vi "SVD_ImagePerEig.vi"(0 "frame":i32, 6 "first N index":i32, 8 "output cluster":T2, 10 "Index Order":dbl[](array[numeric]), 11 "Input Casarati":cdb[][](array[numeric])) -> (2 "StackedImages":cdb[][][](array[numeric]))   [LabVIEW 2022 SP3]
uses:
  <vilib>/Analysis/Matrix/Datatypes/ComplexMatrix.ctl
  <vilib>/Analysis/7linalg.llb/Complex Conjugate Transpose Matrix.vi
  <vilib>/Analysis/baseanly.llb/Complex Outer Product.vi
  <vilib>/Analysis/baseanly.llb/Complex A x B.vi
  <vilib>/Analysis/Matrix/Numeric/Conversions/Matrix To Array - CM.vi
  <vilib>/Analysis/NI_AALPro.lvlib
  <vilib>/Analysis/NI_AALBase.lvlib
  <vilib>/Analysis/Matrix/NI_Matrix.lvlib
panel:
  out "case":i32
  in  "iamge":i32
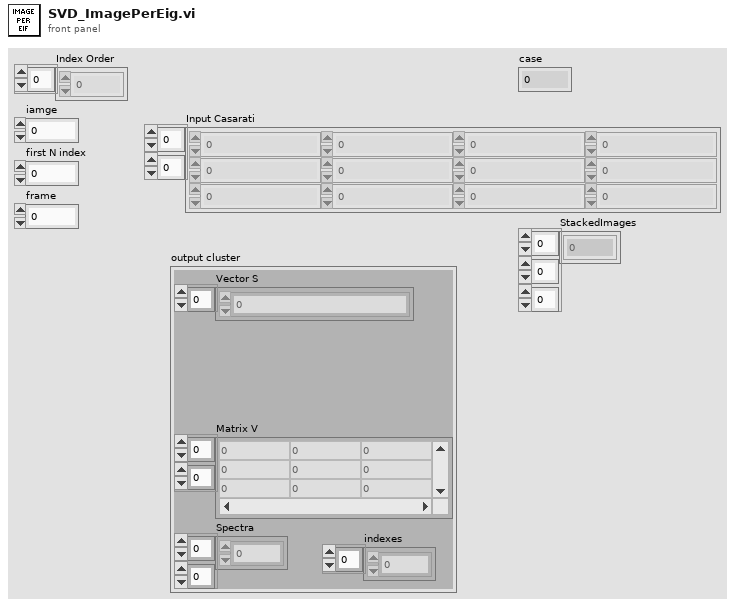
[diagram p1: front panel]
types:
  T1 = typedef "NI_Matrix.lvlib/ComplexMatrix.ctl" = cdb[][]
  T2 = cluster{"Vector S":cdb[], "Matrix V":T1, "Spectra":dbl[][], "indexes":i32[]}
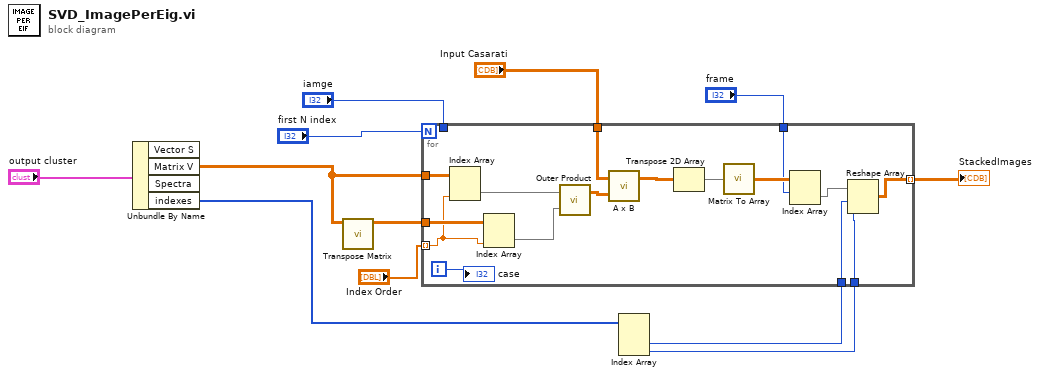
[diagram p0: block diagram]
diagram:
  n1 = Unbundle By Name("output cluster") -> ("Matrix V"=w6:T1, "indexes"=w9:i32[])  [unwired: 2 out]
  n2 = call-poly <vilib>:"Transpose Matrix.vi"("Input Matrix"=w6) -> ("Matrix Conjugate Transpose"=w11:T1)  [unwired: 9 in, 1 out]
  n3 = Index Array(array=w9) -> (element #2=w5:i32, element #3=w4:i32)  [unwired: 3 in, 1 out]
  n4 = for {
    N: "first N index" -> [_]
    tunnel: w6 -> [w28]
    tunnel: w11 -> [w27]
    tunnel: "Input Casarati" -> [w22]
    tunnel: [w15] -> w1 mode=indexing
    tunnel: "Index Order" -> [w26] mode=indexing
    tunnel: "iamge" -> [_]
    tunnel: w5 -> [w17]
    tunnel: w4 -> [w16]
    tunnel: "frame" -> [w13]
    i -> [w14]
    n5 = Index Array(array=w28, index (col)=w26) -> (element=w25:cdb[])  [unwired: 1 in]
    n6 = Index Array(array=w27, index (col)=w26) -> (element=w24:cdb[])  [unwired: 1 in]
    n7 = call-poly <vilib>:"Outer Product.vi"("Y Vector"=w24, "X Vector"=w25) -> ("Outer Product"=w23:T1)  [unwired: 1 out]
    n8 = call-poly <vilib>:"A x B.vi"("B"=w23, "A"=w22) -> ("A x B"=w21:T1)  [unwired: 1 out]
    n9 = Transpose 2D Array(2D array=w21) -> (transposed array=w20:T1)
    n10 = call-poly <vilib>:"Matrix To Array.vi"("Complex Matrix"=w20) -> ("Complex 2D Array"=w19:cdb[][])
    n11 = Index Array(array=w19, index (row)=w13) -> (element=w18:cdb[])  [unwired: 1 in]
    n12 = Reshape Array(w18, w17, w16) -> (w15:cdb[][])
    "case" <- w14
  }
  "StackedImages" <- w1
